vi "app - view -- guided sweep.vi"() -> ()   [LabVIEW 2015]
uses:
  github/resonant_ultrasound_A/maglab ultrasound -- arkady/ctl -- name dispatcher -- action.ctl
  github/resonant_ultrasound_A/maglab ultrasound -- arkady/next chunk - read-write freq PID file - atomic actions .vi
  github/resonant_ultrasound_A/maglab ultrasound -- arkady/ctl -- name dispatcher.vi
  github/resonant_ultrasound_A/maglab ultrasound -- arkady/tale of three indices.vi
  github/resonant_ultrasound_A/maglab ultrasound -- arkady/linear interpolation - real.vi
  github/resonant_ultrasound_A/maglab ultrasound -- arkady/line -- complex.vi
  github/resonant_ultrasound_A/maglab ultrasound -- arkady/Q -- check range -- i -- integer.vi
  github/resonant_ultrasound_A/maglab ultrasound -- arkady/file -- 9w path.vi
  github/resonant_ultrasound_A/maglab ultrasound -- arkady/array -- find index - real.vi
  github/resonant_ultrasound_A/maglab ultrasound -- arkady/array -- interpolate -- i.vi
  github/resonant_ultrasound_A/maglab ultrasound -- arkady/command stack.vi
  github/resonant_ultrasound_A/maglab ultrasound -- arkady/tale of three indices -- check state.vi
  github/resonant_ultrasound_A/maglab ultrasound -- arkady/Q - not nan -- integer.vi
  github/resonant_ultrasound_A/maglab ultrasound -- arkady/Q -- check range -- i -- real.vi
  github/resonant_ultrasound_A/maglab ultrasound -- arkady/Q - not nan -- real.vi
  <vilib>/Utility/libraryn.llb/Check if File or Folder Exists.vi
  github/resonant_ultrasound_A/maglab ultrasound -- arkady/file -- read list of lines.vi
  github/resonant_ultrasound_A/maglab ultrasound -- arkady/parse -- find first line.vi
  github/resonant_ultrasound_A/maglab ultrasound -- arkady/parse -- get list of matches -- numbers.vi
  <vilib>/Utility/file.llb/Write To Spreadsheet File.vi
  <vilib>/Utility/file.llb/Write To Spreadsheet File (string).vi
  <vilib>/gmath/function.llb/Binomial Coefficient.vi
panel:
  out "temperature":dbl=171.28221040729133
  out "x+y":timestamp=timestamp(3520500972.984763 s since 1904-01-01) format="%<%A, %b%d , %I:%M:%S%p>T"
  in  "Time Stamp":timestamp=timestamp(3555695525.368866 s since 1904-01-01) format="%<%A, %b%d , %I:%M:%S%p>T"
  out "Plot: (min)/sweep vs T":cluster{dbl[], dbl[]}[](graph)
  out "Plot: K/sweep vs T":cluster{dbl[], dbl[]}[](graph)
  out "Plot: voltage":cluster{dbl[], dbl[]}[](graph)=[{[5.0, 30.0, 60.0, 100.0], [0.2, 0.3, 0.5, 0.5]}, {array[1000 elements], array[1000 elements]}]
  in  "N":i32(slide)=1000 min=-506096563 max=2129711151 step=1 scale=0.01..1000.0
  in  "Time max":dbl(slide)=6895.4882445737985 min=-506096563.00000006 max=2129711151.0 step=0.010000000000000002 scale=0.01..10000.0 scale format="%#3_3f"
  in  "time min":dbl(slide)=0.01167520658858774 min=-506096563.00000006 max=2129711151.0 step=0.010000000000000002 scale=0.01..1000.0 scale format="%#3_3f"
  in  "divide T by":i32=1
  out "Plot:  dT  vs T":cluster{dbl[], dbl[]}[](graph)
  out "Plot: T slope":cluster{dbl[], dbl[]}[](graph)
  in  "sweep folder path":path=path "E:/Technique/RUS/LSCO/LSCO22_Hayden_S2_polished/4_cooling"
  out "Plot: Temp vs Time":cluster{dbl[], dbl[]}[](graph)=[{[0.0, 300.0, 800.0, 1600.0, 3200.0], [295.0, 200.0, 140.0, 70.0, 5.0]}, {array[1000 elements], array[1000 elements]}]
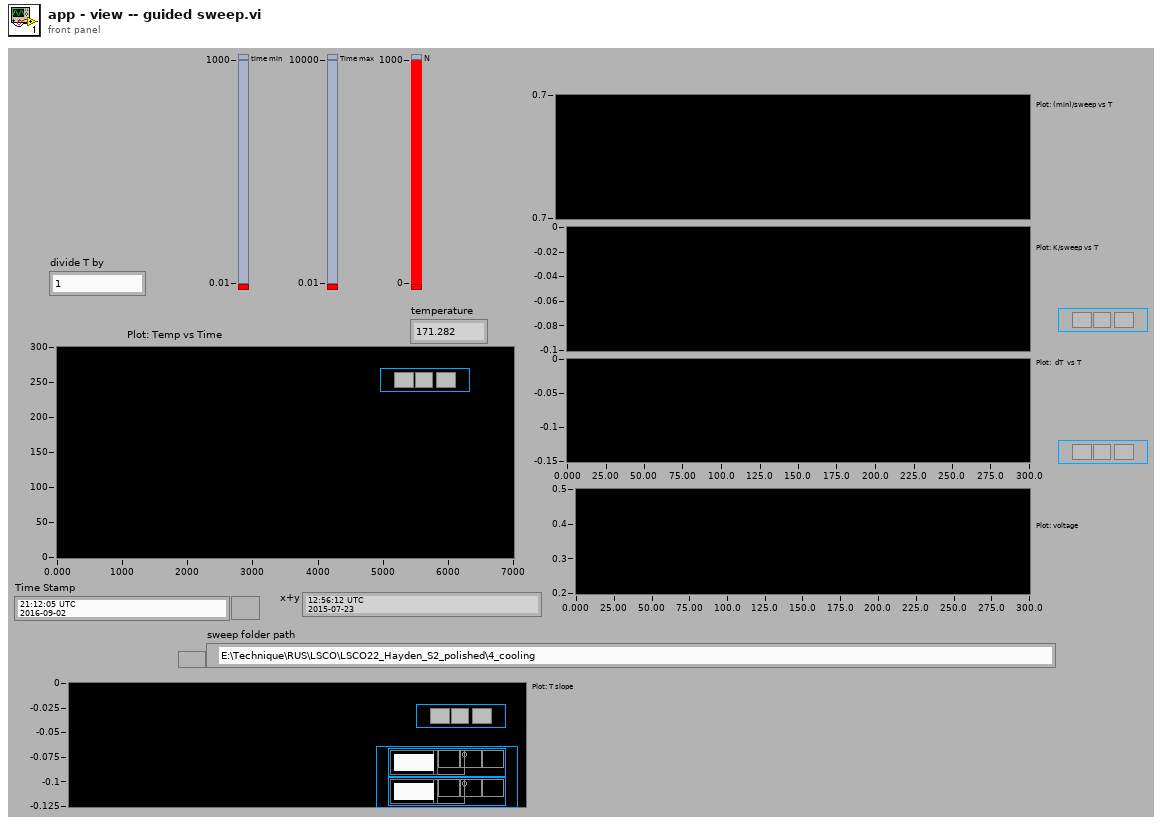
[diagram p1: front panel]
types:
  T1 = typedef "ctl -- name dispatcher -- action.ctl" = enum16{"peak frequency", "peak frequency DUMP", "peak gamma DUMP", "peak gamma", "peak frequency TEST", "peak gamma TEST", "ultrasonic power", "time in gamma", "set temperature ", "set temperature timer", "peak default gamma", "last scan file", "peak freq gamma TEST", "peak NAMES", "errors", "P_I_D", "P", "I", "D", "power vs time", "power vs time TIMER", "void", "power log", "set temperature - SINE", "itc ltc log", "peak - time in gamma"}
  T2 = cluster{"temperatures":dbl[], "frequencies":dbl[]}
  T3 = cluster{"temperatures":dbl[], "frequencies":dbl[]}[]
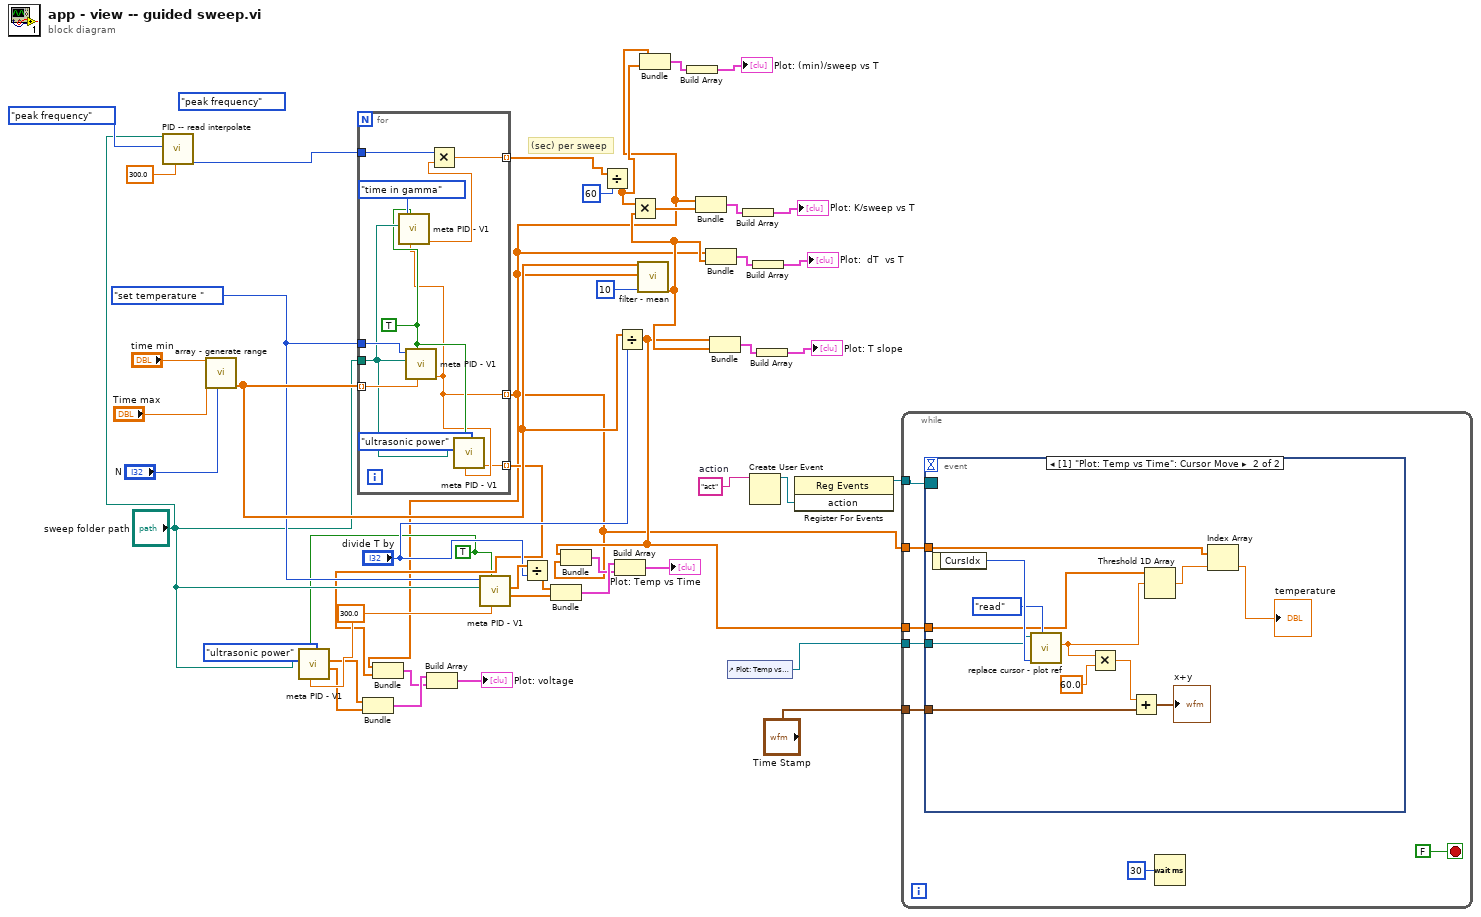
[diagram p0: block diagram]
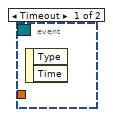
[diagram p2: hidden frame]
diagram:
  w7 = "act"  # action
  (unwired) ctl_--_name_dispatcher_--_action."peak frequency" ("ctl name dispatch")
  w35 = ctl_--_name_dispatcher_--_action."set temperature " ("ctl name dispatch")
  w13 = TRUE ("control power PID?")
  w26 = 300.0 ("nonzero temperature")
  # "(sec) per sweep"
  n1 = call "PID -- read interpolate.vi"("sweep folder path"="sweep folder path", "ctl PID file IN"=ctl_--_name_dispatcher_--_action."peak frequency", "temperature"=300.0) -> ("length out"=w29:i32)  [unwired: 11 in, 5 out]
  n2 = call "array - generate range.vi"("N"="N", "freq max"="Time max", "freq min"="time min") -> ("Array"=w40:dbl[])  [unwired: 7 in, 1 out]
  n3 = call "meta PID - V1.vi"("input parameter"=w26, "control?"=w13, "sweep folder path"="sweep folder path", "ctl name dispatch"=ctl_--_name_dispatcher_--_action."ultrasonic power") -> ("frequencies"=w21:dbl[], "temperatures"=w22:dbl[])  [unwired: 4 in, 2 out]
  n4 = for {
    tunnel: w40 -> [w57] mode=indexing
    tunnel: [w49] -> w1 mode=indexing
    tunnel: "sweep folder path" -> [w51]
    tunnel: w35 -> [w56]
    tunnel: w29 -> [w53]
    tunnel: [w48] -> w20 mode=indexing
    tunnel: [w47] -> w17 mode=indexing
    w50 = TRUE ("control power PID?")
    n5 = call "meta PID - V1.vi"("input parameter"=w57, "control?"=w50, "sweep folder path"=w51, "ctl name dispatch"=w56) -> ("bezier output"=w49:dbl)  [unwired: 4 in, 3 out]
    n6 = call "meta PID - V1.vi"("input parameter"=w49, "control?"=w50, "sweep folder path"=w51, "ctl name dispatch"=ctl_--_name_dispatcher_--_action."time in gamma") -> ("bezier output"=w54:dbl)  [unwired: 4 in, 3 out]
    n7 = Multiply(x=w53, y=w54) -> (x*y=w47:dbl)
    n8 = call "meta PID - V1.vi"("input parameter"=w49, "control?"=w50, "sweep folder path"=w51, "ctl name dispatch"=ctl_--_name_dispatcher_--_action."ultrasonic power") -> ("bezier output"=w48:dbl)  [unwired: 4 in, 3 out]
  }
  n9 = Bundle("temperatures"=w22, "frequencies"=w21) -> (w25:T2)  [unwired: 1 in]
  n10 = Bundle(w1, w20) -> (w24:cluster{dbl[], dbl[]})  [unwired: 1 in]
  n11 = Build Array(w25, w24) -> (→"Plot: voltage":T3)
  n12 = call "meta PID - V1.vi"("input parameter"=w26, "control?"=w13, "sweep folder path"="sweep folder path", "ctl name dispatch"=w35) -> ("frequencies"=w4:dbl[], "temperatures"=w37:dbl[])  [unwired: 4 in, 2 out]
  n13 = Divide(x=w37, y="divide T by") -> (x/y=w3:dbl[])
  n14 = Bundle(w3, "frequencies"=w4) -> (w46:cluster{dbl[], "frequencies":dbl[]})  [unwired: 1 in]
  n15 = Divide(x=w17, y=60) -> (x/y=w10:dbl[])
  n16 = Divide(x=w40, y="divide T by") -> (x/y=w2:dbl[])
  n17 = Bundle(w2, w1) -> (w45:cluster{dbl[], dbl[]})  [unwired: 1 in]
  n18 = Build Array(w46, w45) -> (→"Plot: Temp vs Time":cluster{dbl[], "frequencies":dbl[]}[])
  n19 = call "filter - mean.vi"("omega  in"=w40, "z in"=w1, "window"=10) -> ("slope"=w15:dbl[])  [unwired: 13 in, 3 out]
  n20 = Multiply(x=w10, y=w15) -> (x*y=w14:dbl[])
  n21 = Bundle(w1, w10) -> (w12:cluster{dbl[], dbl[]})  [unwired: 1 in]
  n22 = Build Array(w12) -> (→"Plot: (min)/sweep vs T":cluster{dbl[], dbl[]}[])
  n23 = Bundle(w1, w14) -> (w19:cluster{dbl[], dbl[]})  [unwired: 1 in]
  n24 = Bundle(w1, "slope"=w15) -> (w39:cluster{dbl[], "slope":dbl[]})  [unwired: 1 in]
  n25 = Bundle(w2, "slope"=w15) -> (w43:cluster{dbl[], "slope":dbl[]})  [unwired: 1 in]
  n26 = control-ref of="Plot: Temp vs Time"() -> (w6:refnum<vi>)
  n27 = Build Array(w19) -> (→"Plot: K/sweep vs T":cluster{dbl[], dbl[]}[])
  n28 = Create User Event(user event datatype=w7) -> (user event=w8:refnum<user-event>)  [unwired: 1 in, 1 out]
  n29 = Build Array(w39) -> (→"Plot:  dT  vs T":cluster{dbl[], "slope":dbl[]}[])
  n30 = Build Array(w43) -> (→"Plot: T slope":cluster{dbl[], "slope":dbl[]}[])
  n31 = register-events(w8) -> (reference out=w9:refnum<event-registration>)  [unwired: 2 in, 1 out]
  n32 = while {
    tunnel: w9 -> [w64]
    tunnel: w6 -> [w63]
    tunnel: "Time Stamp" -> [w60]
    tunnel: w1 -> [w59]
    tunnel: w2 -> [w58]
    stop <- FALSE stop-if-true
    n33 = event shown="[1] \"Plot: Temp vs Time\": Cursor Move" {
      selector: w64 -> [_ _]
      dyn-events: _ -> [_ _]
      timeout: _ -> [_ _]
      tunnel: w63 -> [_ w75]
      tunnel: w60 -> [_ w71]
      tunnel: w59 -> [_ w66]
      tunnel: w58 -> [_ w68]
      event Timeout {
        n34 = event-data() -> ()  [unwired: 1 in, 2 out]
      }
      event "Plot: Temp vs Time": Cursor Move {
        n35 = event-data() -> ("CursIdx"=w76:i32)  [unwired: 1 in]
        n36 = call "replace cursor - plot ref.vi"("action"=enum16{"", "read", "write"}."read", "cursor index"=w76, "Plot ref in"=w75) -> ("read X"=w69:dbl)  [unwired: 6 in, 2 out]
        n37 = Multiply(x=w69, y=60.0) -> (x*y=w72:dbl)
        n38 = Add(x=w72, y=w71) -> (x+y=→"x+y":timestamp)
        n39 = Threshold 1D Array(2:w69, 3:w68) -> (0:w67:dbl)  [unwired: 1 in]
        n40 = Index Array(array=w66, index=w67) -> (element=→"temperature":dbl)
      }
    }
    n41 = Wait (ms)(milliseconds to wait=u32 30) -> ()  [unwired: 1 out]
  }
